vi "ref Begin.vi"(8 "error in":errorcluster) -> (0 "error out":errorcluster)   [LabVIEW 2020]
doc: "Called before other user functions, this VI is expected to open initial I/O refnums, load in file data, and do all program initialization. Notice that the <B>error out</B> terminal is simply used for data flow. Wiring it to other structures or subVIs ensures that this VI runs first."
uses:
  <vilib>/Rock Robotics/WPI/ThirdParty/Phoenix-LabVIEW/Motor Controller/Controls/CTRE_Phoenix_MotorControl_TalonFXMotorControllerConfigurables.ctl
  <vilib>/Rock Robotics/WPI/ThirdParty/Phoenix-LabVIEW/Motor Controller/Controls/CTRE_Phoenix_MotorControl_BaseConfigurables.ctl
  <vilib>/Rock Robotics/WPI/ThirdParty/Phoenix-LabVIEW/Motor Controller/Controls/CTRE_Phoenix_MotorControl_VelocityMeasurementPeriod.ctl
  <vilib>/Rock Robotics/WPI/ThirdParty/Phoenix-LabVIEW/Motor Controller/Controls/CTRE_Phoenix_MotorControl_SlotStructure.ctl
  <vilib>/Rock Robotics/WPI/ThirdParty/Phoenix-LabVIEW/Motor Controller/Controls/CTRE_Phoenix_MotorControl_FilterStruct.ctl
  <vilib>/Rock Robotics/WPI/ThirdParty/Phoenix-LabVIEW/Motor Controller/Controls/CTRE_Phoenix_MotorControl_RemoteSourceType.ctl
  <vilib>/Rock Robotics/WPI/ThirdParty/Phoenix-LabVIEW/Controls/CTRE_Phoenix_CustomParamConfiguration.ctl
  <vilib>/Rock Robotics/WPI/ThirdParty/Phoenix-LabVIEW/Motor Controller/Controls/CTRE_Phoenix_MotorControl_FeedbackDevice_TalonFX.ctl
  <vilib>/Rock Robotics/WPI/ThirdParty/Phoenix-LabVIEW/Motor Controller/Controls/CTRE_Phoenix_MotorControl_LimitSwitchNormal.ctl
  <vilib>/Rock Robotics/WPI/ThirdParty/Phoenix-LabVIEW/Motor Controller/Controls/CTRE_Phoenix_MotorControl_LimitSwitchSource_Local.ctl
  <vilib>/Rock Robotics/WPI/ThirdParty/Phoenix-LabVIEW/Motor Controller/Controls/CTRE_Phoenix_MotorControl_SupplyCurrentLimitConfiguration.ctl
  <vilib>/Rock Robotics/WPI/ThirdParty/Phoenix-LabVIEW/Motor Controller/Controls/CTRE_Phoenix_MotorControl_StatorCurrentLimitConfiguration.ctl
  <vilib>/Rock Robotics/WPI/ThirdParty/Phoenix-LabVIEW/Motor Controller/Controls/CTRE_Phoenix_MotorControl_MotorCommutation_TalonFX.ctl
  <vilib>/Rock Robotics/WPI/ThirdParty/Phoenix-LabVIEW/CANCoder/Controls/CTRE_Phoenix_CANcoder_AbsoluteSensorRange.ctl
  <vilib>/Rock Robotics/WPI/ThirdParty/Phoenix-LabVIEW/CANCoder/Controls/CTRE_Phoenix_CANcoder_SensorInitializationStrategy.ctl
  <vilib>/Rock Robotics/WPI/ThirdParty/Phoenix-LabVIEW/Motor Controller/Controls/CTRE_Phoenix_MotorControl_NeutralMode.ctl
  <vilib>/Rock Robotics/SystemInterfaces/DIO/FPGA_DIOChannel.ctl
  <vilib>/Rock Robotics/SystemInterfaces/DIO/FPGA_DIOPWMChannel.ctl
  <vilib>/Rock Robotics/WPI/Joystick/WPI_Joystick Info.ctl
  <vilib>/Rock Robotics/WPI/Joystick/WPI_JoystickHID Types.ctl
  <vilib>/Rock Robotics/WPI/Joystick/WPI_JoystickXBox Types.ctl
  <vilib>/Rock Robotics/WPI/Joystick/WPI_JoystickAxis Types.ctl
  <vilib>/Rock Robotics/WPI/Ultrasonic/WPI_UltrasonicRangeUnits.ctl
  <vilib>/Rock Robotics/WPI/Joystick/WPI_JoystickDeviceEnum.ctl
  <vilib>/Rock Robotics/WPI/DriverStation/WPI_DriverStationRobotMode2.ctl
  <vilib>/Rock Robotics/WPI/SafetyOutput/WPI_SafetyOutputConfigMenu.ctl
  <vilib>/Rock Robotics/SystemInterfaces/AI/FPGA_AIChannel.ctl
  <vilib>/Rock Robotics/SystemInterfaces/i2clib/i2c_bus.ctl
  <vilib>/Rock Robotics/Network Tables/NT Write String Array.vi
  Robot Global Data.vi
  <vilib>/Rock Robotics/WPI/RobotDrive/WPI_RobotDriveOpen2MotorWithExistingMotors.vi
  <vilib>/Rock Robotics/WPI/ThirdParty/REV Robotics/REVLib/Typedef/Spark MAX Motor Type.ctl
  <vilib>/Rock Robotics/WPI/ThirdParty/REV Robotics/REVLib/Typedef/Spark MAX Idle Mode.ctl
  <vilib>/Rock Robotics/Network Tables/NT Write Number.vi
  <vilib>/Rock Robotics/WPI/Ultrasonic/WPI_SonarSRF04DigitalOpen.vi
  <vilib>/Rock Robotics/WPI/Ultrasonic/WPI_SonarSRF04DigitalRefNum Registry Set.vi
  <vilib>/Rock Robotics/WPI/Ultrasonic/WPI_SonarSRF04DigitalGetRange.vi
  <vilib>/Rock Robotics/WPI/Counter/WPI_CounterDigitalInputToDigitalSource.vi
  <vilib>/Rock Robotics/Network Tables/NT Write Boolean.vi
  <vilib>/Rock Robotics/WPI/Counter/WPI_CounterOpen Gear Tooth Sensor Mode.vi
panel:
  in  "KICKER CAN ID 2":u8=10
  in  "Tab Control":T1(tab)=enum."SHOOTER"
  in  "drive wheel diameter (in)":dbl=6.0 format="%.3g"
  in  "drive gearbox ratio":dbl=10.71
  out "wheel circumference":dbl=18.84955592153876
  in  "MASTER LEFT DRIVE CAN ID":u8=2
  in  "LEFT MotorInverted":bool=TRUE
  in  "Motor Control Neutral Mode 3":T2=enum."Override to Coast"
  in  "CLIMBER COAST":T2=enum."Override to Brake"
  in  "CLIMBER LEFT CAN ID":u8=9
  in  "ARM LEFT CAN ID":u8=11
  in  "CLIMBER RIGHT CAN ID":u8=7
  in  "ARM RIGHT CAN ID":u8=15
  in  "Invert LEFT climber":bool
  in  "Invert arm actuators":bool
  in  "FALCON shooter config":T3={"Base Configurables"={"openLoopRamp"=0.0, "closedLoopRamp"=0.0, "peakOutputForward"=1.0, "peakOutputReverse"=-1.0, "nominalOutputForward"=0.0, "nominalOutputReverse"=0.0, "neutralDeadband"=0.04, "voltageCompSaturation"=0.0, "voltageMeasurementFilter"=32, "velocityMeasurementPeriod"=100, "velocityMeasurementWindow"=64, "forwardSoftLimitThreshold"=0, "reverseSoftLimitThreshold"=0, "forwardSoftLimitEnable"=FALSE, "reverseSoftLimitEnable"=FALSE, "slot0"={"P"=0.0, "I"=0.0, "D"=0.0, "F"=0.0, "integralZone"=0.0, "allowableClosedLoopError"=0, "maxIntegralAccumulator"=0.0, "closedLoopPeakOutput"=1.0, "closedLoopPeriod"=1}, "slot1"={"P"=0.0, "I"=0.0, "D"=0.0, "F"=0.0, "integralZone"=0.0, "allowableClosedLoopError"=0, "maxIntegralAccumulator"=0.0, "closedLoopPeakOutput"=1.0, "closedLoopPeriod"=1}, "slot2"={"P"=0.0, "I"=0.0, "D"=0.0, "F"=0.0, "integralZone"=0.0, "allowableClosedLoopError"=0, "maxIntegralAccumulator"=0.0, "closedLoopPeakOutput"=1.0, "closedLoopPeriod"=1}, "slot3"={"P"=0.0, "I"=0.0, "D"=0.0, "F"=0.0, "integralZone"=0.0, "allowableClosedLoopError"=0, "maxIntegralAccumulator"=0.0, "closedLoopPeakOutput"=1.0, "closedLoopPeriod"=1}, "auxPIDPolarity"=FALSE, "remoteFilter0"={"remoteSensorDeviceID"=0, "remoteSensorSource"=enum."Off"}, "remoteFilter1"={"remoteSensorDeviceID"=0, "remoteSensorSource"=enum."Off"}, "motionCruiseVelocity"=0, "motionAcceleration"=0, "motionProfileTrajectoryPeriod"=0, "feedbackNotContinuous"=FALSE, "remoteSensorClosedLoopDisableNeutralOnLOS"=FALSE, "clearPositionOnLimitF"=FALSE, "clearPositionOnLimitR"=FALSE, "clearPositionOnQuadIdx"=FALSE, "limitSwitchDisableNeutralOnLOS"=FALSE, "softLimitDisableNeutralOnLOS"=FALSE, "pulseWidthPeriod_EdgesPerRot"=1, "pulseWidthPeriod_FilterWindowSz"=1, "customParam"={"customParam0"=0, "customParam1"=0}, "trajectoryInterpolationEnable"=TRUE}, "primaryPID"={"selectedFeedbackCoefficient"=1.0, "selectedFeedbackSensor"=1}, "auxiliaryPID"={"selectedFeedbackCoefficient"=1.0, "selectedFeedbackSensor"=1}, "forwardLimitSwitchNormal"=enum."Normally Open", "reverseLimitSwitchNormal"=enum."Normally Open", "forwardLimitSwitchDeviceID"=0, "reverseLimitSwitchDeviceID"=0, "forwardLimitSwitchSource"=enum."Feedback Connector", "reverseLimitSwitchSource"=enum."Feedback Connector", "sum0Term"=1, "sum1Term"=1, "diff0Term"=1, "diff1Term"=1, "Supply Current Limit Configuration"={"Enable?"=FALSE, "Current Limit"=0.0, "Threshold Current"=0.0, "Threshold Time"=0.0}, "Stator Current Limit Configuration"={"Enable?"=FALSE, "Current Limit"=0.0, "Threshold Current"=0.0, "Threshold Time"=0.0}, "Motor Commutation"=enum."Trapezoidal", "Absolute Sensor Range"=enum."Unsigned [0 to 360)", "Integrated Sensor Offset (Degrees)"=0.0, "Sensor Initialization Strategy"=enum."Boot To Zero"} {"diff1Term" items=["Integrated Sensor"=1, "Sensor Sum (S0 + S1)"=9, "Sensor Difference (D0 - D1)"=10, "Remote Source 0"=11, "Remote Source 1"=12, "None"=14, "Software Emulated"=15]; "diff0Term" items=["Integrated Sensor"=1, "Sensor Sum (S0 + S1)"=9, "Sensor Difference (D0 - D1)"=10, "Remote Source 0"=11, "Remote Source 1"=12, "None"=14, "Software Emulated"=15]; "sum1Term" items=["Integrated Sensor"=1, "Sensor Sum (S0 + S1)"=9, "Sensor Difference (D0 - D1)"=10, "Remote Source 0"=11, "Remote Source 1"=12, "None"=14, "Software Emulated"=15]; "sum0Term" items=["Integrated Sensor"=1, "Sensor Sum (S0 + S1)"=9, "Sensor Difference (D0 - D1)"=10, "Remote Source 0"=11, "Remote Source 1"=12, "None"=14, "Software Emulated"=15]; "auxiliaryPID"."selectedFeedbackSensor" items=["Integrated Sensor"=1, "Sensor Sum (S0 + S1)"=9, "Sensor Difference (D0 - D1)"=10, "Remote Source 0"=11, "Remote Source 1"=12, "None"=14, "Software Emulated"=15]; "primaryPID"."selectedFeedbackSensor" items=["Integrated Sensor"=1, "Sensor Sum (S0 + S1)"=9, "Sensor Difference (D0 - D1)"=10, "Remote Source 0"=11, "Remote Source 1"=12, "None"=14, "Software Emulated"=15]; "Base Configurables"."velocityMeasurementPeriod" items=["Period_1ms"=1, "Period_2ms"=2, "Period_5ms"=5, "Period_10ms"=10, "Period_20ms"=20, "Period_25ms"=25, "Period_50ms"=50, "Period_100ms"=100]}
  in  "Motor Control Neutral Mode 2":T2=enum."Override to Brake"
  in  "SHOOTER CAN ID":u8=8
  in  "KICKER CAN ID":u8=21
  in  "KICKER COUNT DIO":T18
  in  "Sonars":T20(array[cluster])=[{"Sonar refnum name"="BALL1", "Ping DIO Channel"=enum."DIO 2", "Echo DIO Channel"=enum."DIO 3", "Range Units"=enum."inches"}, {"Sonar refnum name"="BALL2", "Ping DIO Channel"=enum."DIO 4", "Echo DIO Channel"=enum."DIO 5", "Range Units"=enum."inches"}]
  in  "Color Define":T21(array[cluster])
  out "Joystick INFO":T22[](array[typedef])
  in  "Joysticks":T27(array[cluster])=[{"JoystickDevice"=enum."USB 0", "refnum name"="Joystick 0"}, {"JoystickDevice"=enum."USB 1", "refnum name"="Joystick LEFT"}, {"JoystickDevice"=enum."USB 2", "refnum name"="Joystick RIGHT"}]
  in  "Power Distribution (def)":u8
  in  "Clear Sticky Faults":bool
  out "Channel Faults":bool[](array[boolean])
  out "Faults":T28
  out "Sticky Faults":T29
  out "error out 2":errorcluster={"status"=TRUE, "code"=-44087, "source"="NetComm_CAN_Receive.vi:5470010<APPEND>\n\n<b>Complete call chain:</b>\n     NetComm_CAN_Receive.vi:5470010\n     WPI_CAN_PDHReceive.vi\n     WPI_Power Get PD Faults.vi\n     Begin.vi\n     Robot Main.vi"}
  in  "TILT zero":u16=68
  in  "TILT Range":u16=170
  in  "PAN zero":u16=85
  in  "TILT  PWM Channel":T30=enum."PWM 1"
  in  "PAN Range":u16=170
  in  "PAN PWM Channel":T30
  # "Sum and Diff terms are ways to select more than one sensor as a feedback device. \n Sum 0 is the first feedback device to be used for the Sum term.\n Sum 1 is the feedback device to be added to Sum 0 for the Sum term.\n Diff 0 and Diff 1 work in a similar manner."
  # "These are only applicable\nif using a remote limit switch.\n\nLocal limit switches/no limit\nswitches do not use this."
  # "Current is below Current Limit AND\n\n(Requested output is weaker** than applied motor\noutput OR is in the opposite direction).\n/\nMotor output is set to requested output."
  # "Current is above Threshold Current for Threshold Time\n/\nReduce motor output (towards neutral)."
  # "Current is below Current Limit.\n/\nRamp motor output towards requested output."
  # "Current is above Current Limit.\n/\nReduce motor output (towards neutral)."
  # "*If the configured Peak Threshold is less than the Continuous Threshold, the applied Peak Threshold is set equal to the Configured Continuous Threshold in firmware.\n** Both requested output and applied motor output are in the same direction, and requested output is closer to neutral."
  # "False: Primary Output = PID[0] + PID[1]  ---  Auxiliary Output = PID[0] - PID[1]\nTrue:  Primary Output = PID[0] - PID[1] --- Auxiliary Output = PID[0] + PID[1]"
  # "Enable the motion profile executor to perform linear interpolation between profile points.  Defaults to True."
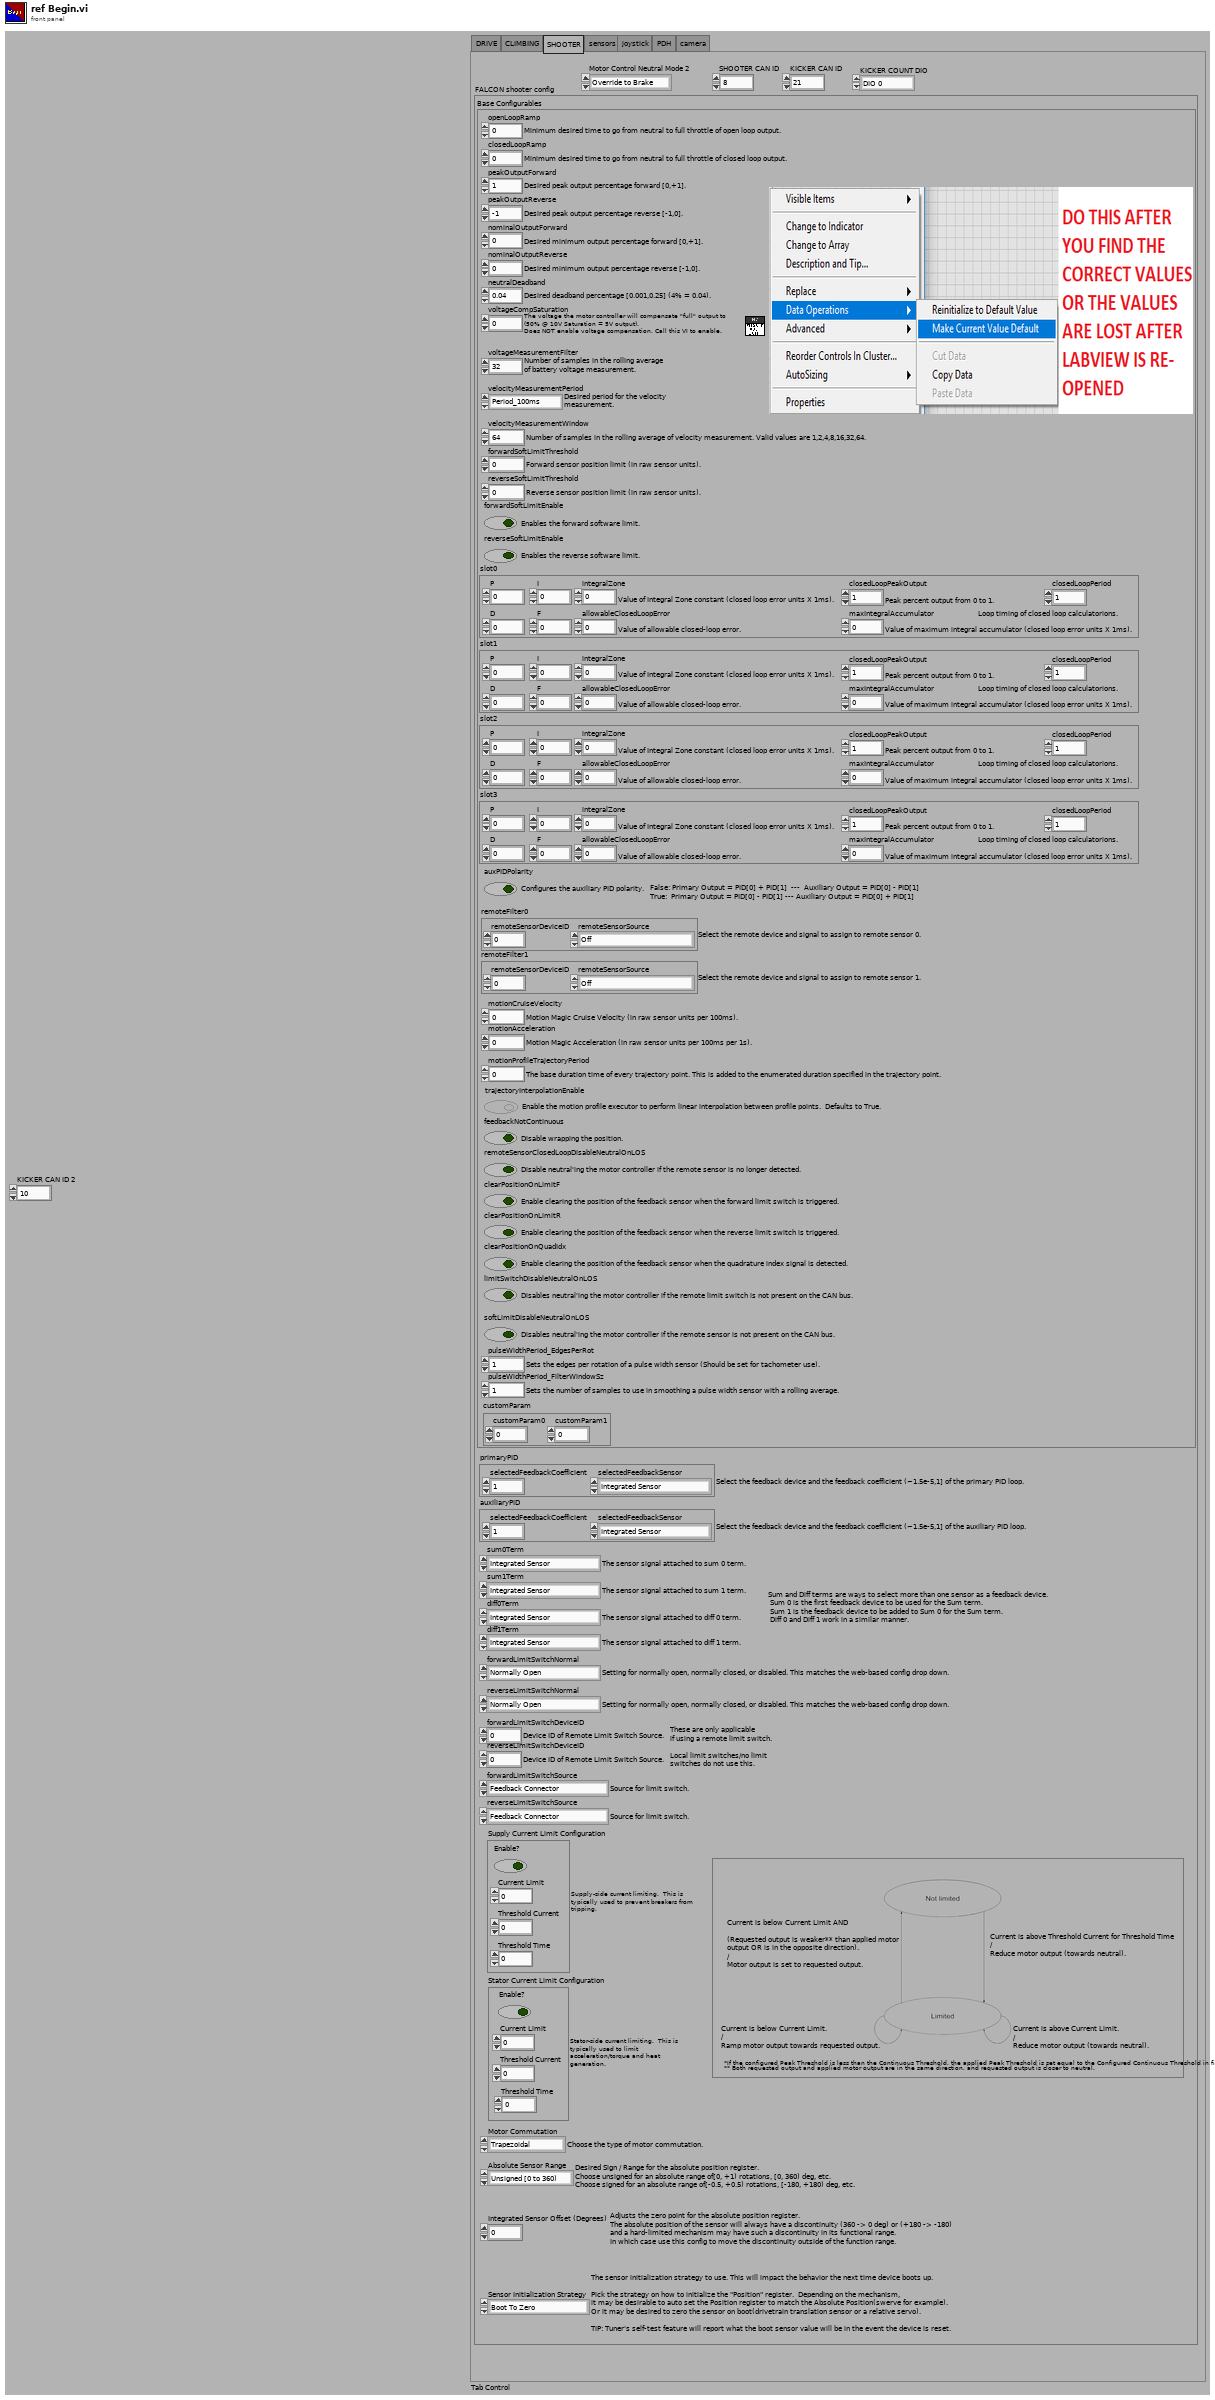
[diagram p1: front panel]
types:
  T1 = enum32{"DRIVE", "CLIMBING", "SHOOTER", "sensors", "joystick", "PDH", "camera"}
  T2 = typedef "CTRE_Phoenix_MotorControl_NeutralMode.ctl" = enum8{"EEPROMSetting", "Override to Coast", "Override to Brake"}
  T3 = typedef "CTRE_Phoenix_MotorControl_TalonFXMotorControllerConfigurables.ctl" = cluster{"Base Configurables":T4, "primaryPID":cluster{"selectedFeedbackCoefficient":dbl, "selectedFeedbackSensor":T10}, "auxiliaryPID":cluster{"selectedFeedbackCoefficient":dbl, "selectedFeedbackSensor":T10}, "forwardLimitSwitchNormal":T11, "reverseLimitSwitchNormal":T11, "forwardLimitSwitchDeviceID":i32, "reverseLimitSwitchDeviceID":i32, "forwardLimitSwitchSource":T12, "reverseLimitSwitchSource":T12, "sum0Term":T10, "sum1Term":T10, "diff0Term":T10, "diff1Term":T10, "Supply Current Limit Configuration":T13, "Stator Current Limit Configuration":T14, "Motor Commutation":T15, "Absolute Sensor Range":T16, "Integrated Sensor Offset (Degrees)":dbl, "Sensor Initialization Strategy":T17}
  T4 = typedef "CTRE_Phoenix_MotorControl_BaseConfigurables.ctl" = cluster{"openLoopRamp":dbl, "closedLoopRamp":dbl, "peakOutputForward":dbl, "peakOutputReverse":dbl, "nominalOutputForward":dbl, "nominalOutputReverse":dbl, "neutralDeadband":dbl, "voltageCompSaturation":dbl, "voltageMeasurementFilter":i32, "velocityMeasurementPeriod":T5, "velocityMeasurementWindow":i32, "forwardSoftLimitThreshold":i32, "reverseSoftLimitThreshold":i32, "forwardSoftLimitEnable":bool, "reverseSoftLimitEnable":bool, "slot0":T6, "slot1":T6, "slot2":T6, "slot3":T6, "auxPIDPolarity":bool, "remoteFilter0":T7, "remoteFilter1":T7, "motionCruiseVelocity":i32, "motionAcceleration":i32, "motionProfileTrajectoryPeriod":i32, "feedbackNotContinuous":bool, "remoteSensorClosedLoopDisableNeutralOnLOS":bool, "clearPositionOnLimitF":bool, "clearPositionOnLimitR":bool, "clearPositionOnQuadIdx":bool, "limitSwitchDisableNeutralOnLOS":bool, "softLimitDisableNeutralOnLOS":bool, "pulseWidthPeriod_EdgesPerRot":i32, "pulseWidthPeriod_FilterWindowSz":i32, "customParam":T9, "trajectoryInterpolationEnable":bool}
  T5 = typedef "CTRE_Phoenix_MotorControl_VelocityMeasurementPeriod.ctl" = u16
  T6 = typedef "CTRE_Phoenix_MotorControl_SlotStructure.ctl" = cluster{"P":dbl, "I":dbl, "D":dbl, "F":dbl, "integralZone":dbl, "allowableClosedLoopError":i32, "maxIntegralAccumulator":dbl, "closedLoopPeakOutput":dbl, "closedLoopPeriod":i32}
  T7 = typedef "CTRE_Phoenix_MotorControl_FilterStruct.ctl" = cluster{"remoteSensorDeviceID":u8, "remoteSensorSource":T8}
  T8 = typedef "CTRE_Phoenix_MotorControl_RemoteSourceType.ctl" = enum16{"Off", "Talon SRX Selected Sensor", "Pigeon IMU Yaw", "Pigeon IMU Pitch", "Pigeon IMU Roll", "CANifier Quadrature", "CANifier PWM Input 0", "CANifier PWM Input 1", "CANifier PWM Input 2", "CANifier PWM Input 3", "Gadgeteer Pigeon Yaw", "Gadgeteer Pigeon Pitch", "Gadgeteer Pigeon Roll", "CANCoder"}
  T9 = typedef "CTRE_Phoenix_CustomParamConfiguration.ctl" = cluster{"customParam0":i32, "customParam1":i32}
  T10 = typedef "CTRE_Phoenix_MotorControl_FeedbackDevice_TalonFX.ctl" = i8
  T11 = typedef "CTRE_Phoenix_MotorControl_LimitSwitchNormal.ctl" = enum16{"Normally Open", "Normally Closed", "Disabled"}
  T12 = typedef "CTRE_Phoenix_MotorControl_LimitSwitchSource_Local.ctl" = enum16{"Feedback Connector", "Remote Talon SRX", "Remote CANifier", "Deactivated"}
  T13 = typedef "CTRE_Phoenix_MotorControl_SupplyCurrentLimitConfiguration.ctl" = cluster{"Enable?":bool, "Current Limit":dbl, "Threshold Current":dbl, "Threshold Time":dbl}
  T14 = typedef "CTRE_Phoenix_MotorControl_StatorCurrentLimitConfiguration.ctl" = cluster{"Enable?":bool, "Current Limit":dbl, "Threshold Current":dbl, "Threshold Time":dbl}
  T15 = typedef "CTRE_Phoenix_MotorControl_MotorCommutation_TalonFX.ctl" = enum16{"Trapezoidal"}
  T16 = typedef "CTRE_Phoenix_CANcoder_AbsoluteSensorRange.ctl" = enum16{"Unsigned [0 to 360)", "Signed [-180 to +180)"}
  T17 = typedef "CTRE_Phoenix_CANcoder_SensorInitializationStrategy.ctl" = enum16{"Boot To Zero", "Boot To Absolute Position"}
  T18 = typedef "FPGA_DIOChannel.ctl" = enum8{"DIO 0", "DIO 1", "DIO 2", "DIO 3", "DIO 4", "DIO 5", "DIO 6", "DIO 7", "DIO 8", "DIO 9", "DIO MXP 0", "DIO MXP 1", "DIO MXP 2", "DIO MXP 3", "DIO MXP 4", "DIO MXP 5", "DIO MXP 6", "DIO MXP 7", "DIO MXP 8", "DIO MXP 9", "DIO MXP 10", "DIO MXP 11", "DIO MXP 12", "DIO MXP 13", "DIO MXP 14", "DIO MXP 15", "SPI Port CS1", "SPI Port CS2", "SPI Port CS3", "SPI Port MISO", "SPI Port MOSI", "Invalid"}
  T19 = typedef "WPI_UltrasonicRangeUnits.ctl" = enum16{"inches", "mm"}
  T20 = cluster{"Sonar refnum name":string, "Ping DIO Channel":T18, "Echo DIO Channel":T18, "Range Units":T19}[]
  T21 = cluster{"Name":string, "Color":cluster{"R":dbl, "G":dbl, "B":dbl}}[]
  T22 = typedef "WPI_Joystick Info.ctl" = cluster{"Device Name":string, "HID Type":T23, "XBox Type":T24, "Axes Count":i32, "Axes Types":T25[], "Button Count":i32, "POV Count":i32}
  T23 = typedef "WPI_JoystickHID Types.ctl" = enum16{"Not HID", "HID Joystick", "HID Gamepad", "HID Driving Wheel", "HID Flightstick", "HID First Person"}
  T24 = typedef "WPI_JoystickXBox Types.ctl" = enum16{"Not XBox", "XBox Unknown", "XBox Gamepad", "XBox Wheel", "XBox Arcade Stick", "XBox Flight Stick", "XBox Dance Pad", "XBox Guitar", "XBox Drum Kit", "XBox Arcade Pad"}
  T25 = typedef "WPI_JoystickAxis Types.ctl" = enum16{"X Axis", "Y Axis", "Z Axis", "RxAxis", "RyAxis", "RzAxis", "Slider", "POV", "None", "L X Axis", "L Y Axis", "L Trigger", "R Trigger", "R X Axis", "R Y Axis"}
  T26 = typedef "WPI_JoystickDeviceEnum.ctl" = enum16{"USB 0", "USB 1", "USB 2", "USB 3", "USB 4", "USB 5"}
  T27 = cluster{"JoystickDevice":T26, "refnum name":string}[]
  T28 = cluster{"Battery Voltage Fault":bool, "Hardware Fault":bool, "CAN Warning Fault":bool, "Temperature Fault":bool}
  T29 = cluster{"Brownout":bool, "CAN Warning":bool, "Can Bus Off":bool, "Hardware Fault":bool, "Firmware Fault":bool, "CH20 Brownout":bool, "CH21 Brownout":bool, "CH22 Brownout":bool, "CH23 Brownout":bool, "Has Reset":bool}
  T30 = typedef "FPGA_DIOPWMChannel.ctl" = enum8{"PWM 0", "PWM 1", "PWM 2", "PWM 3", "PWM 4", "PWM 5", "PWM 6", "PWM 7", "PWM 8", "PWM 9", "PWM MXP 0", "PWM MXP 1", "PWM MXP 2", "PWM MXP 3", "PWM MXP 4", "PWM MXP 5", "PWM MXP 6", "PWM MXP 7", "PWM MXP 8", "PWM MXP 9", "Invalid"}
  T31 = typedef "WPI_ServoDeviceRef.ctl" = cluster{"DeviceStatus":errorcluster, "PWM Channel":T30, "DeadBand":T32}
  T32 = typedef "WPI_PWMDeadband.ctl" = cluster{"Name":string, "maxPositivePwm":i32, "minPositivePwm":i32, "centerPwm":i32, "maxNegativePwm":i32, "minNegativePwm":i32, "angularRange":u16}
  T33 = typedef "WPI_MotorControlDeviceRef.ctl" = cluster{"DeviceStatus":errorcluster, "Type":T34, "PWM":cluster{"PWM Channel":T30, "DeadBand":T32}, "CAN":cluster{"Device Number":u8, "SetOutput VI Ref":variant, "GetOutput VI Ref":variant, "Enable VI Ref":variant, "Disable VI Ref":variant, "Data":variant}, "Invert":bool, "DIO PWM":cluster{"PWM \"Enable\" Channel":T30, "DIOChannel":T18, "PWM Rate":dbl}}
  T34 = typedef "WPI_MotorControlType.ctl" = enum16{"PWM", "CAN", "DIO PWM"}
  T35 = typedef "WPI_DriverStationRobotMode2.ctl" = enum16{"Autonomous Disabled", "Autonomous Enabled", "Teleop Disabled", "Teleop Enabled", "Disconnected", "Finish", "Test Disabled", "Test Enabled", "Emergency Stopped"}
  T36 = typedef "WPI_SafetyOutputConfigMenu.ctl" = enum16{"Enable", "Disable"}
  T37 = typedef "WPI_RobotDriveDevRef.ctl" = cluster{"DevStatus":errorcluster, "Motors[]":T33[], "Square Inputs":bool, "Max Output":dbl}
  T38 = typedef "Spark MAX Idle Mode.ctl" = enum16{"Coast", "Brake"}
  T39 = typedef "Spark MAX Motor Type.ctl" = enum16{"Brushed", "Brushless"}
  T40 = typedef "WPI_DigitalInputDevRef.ctl" = cluster{"DevStatus":errorcluster, "DIO Channel":T18}
  T41 = typedef "FPGA_CounterEncoderSourceConvertionLVSourceType.ctl" = cluster{"DevStatus":errorcluster, "AnalogTriggerMode?":bool, "DigitalMode":cluster{"DIO Channel":T42}, "AnalogTriggerMode":cluster{"AnalogTriggerIndex":T43, "OutputType":T44}}
  T42 = typedef "FPGA_DIODigitalSourceChannel.ctl" = enum8{"DIO 0", "DIO 1", "DIO 2", "DIO 3", "DIO 4", "DIO 5", "DIO 6", "DIO 7", "DIO 8", "DIO 9", "DIO MXP 0", "DIO MXP 1", "DIO MXP 2", "DIO MXP 3", "DIO MXP 4", "DIO MXP 5", "DIO MXP 6", "DIO MXP 7", "DIO MXP 8", "DIO MXP 9", "DIO MXP 10", "DIO MXP 11", "DIO MXP 12", "DIO MXP 13", "DIO MXP 14", "DIO MXP 15", "SPI Port CS1", "SPI Port CS2", "SPI Port CS3", "SPI Port MISO", "SPI Port MOSI", "Disabled"}
  T43 = typedef "FPGA_AnalogTriggerIndex.ctl" = enum8{"Trig 0", "Trig 1", "Trig 2", "Trig 3", "Trig 4", "Trig 5", "Trig 6", "Trig 7", "Invalid"}
  T44 = typedef "FPGA_AnalogTriggerOutType.ctl" = enum16{"InWindow", "TriggerState", "Rising", "Falling"}
  T45 = typedef "WPI_CounterDevRef.ctl" = cluster{"DevStatus":errorcluster, "CntIndex":T46}
  T46 = typedef "FPGA_CounterCtrSystemIndex.ctl" = enum8{"Ctr 0", "Ctr 1", "Ctr 2", "Ctr 3", "Ctr 4", "Ctr 5", "Ctr 6", "Ctr 7", "Invalid"}
  T47 = typedef "i2c_bus.ctl" = enum16{"I2C On-Board", "I2C MXP", "Invalid"}
  T48 = typedef "WPI_UltrasonicDeviceRef.ctl" = cluster{"DevStatus":errorcluster, "Ping Channel":T18, "Echo Channel":T18, "CntIndex":T46}
  T49 = typedef "Color Sensor V3 DevRef.ctl" = cluster{"I2CDevRef":T50}
  T50 = typedef "WPI_I2CDevRef.ctl" = cluster{"DevStatus":errorcluster, "Device Address":u8, "Handle":i32, "I2C Bus":T47}
  T51 = typedef "WPI_JoystickDevRef.ctl" = cluster{"Device":T26}
  T52 = typedef "FPGA_AIChannel.ctl" = enum8{"AI 0", "AI 1", "AI 2", "AI 3", "AI MXP 0", "AI MXP 1", "AI MXP 2", "AI MXP 3", "Invalid"}
  T53 = typedef "WPI_AnalogChannelDevRef.ctl" = cluster{"DevStatus":errorcluster, "Analog Channel":T52}
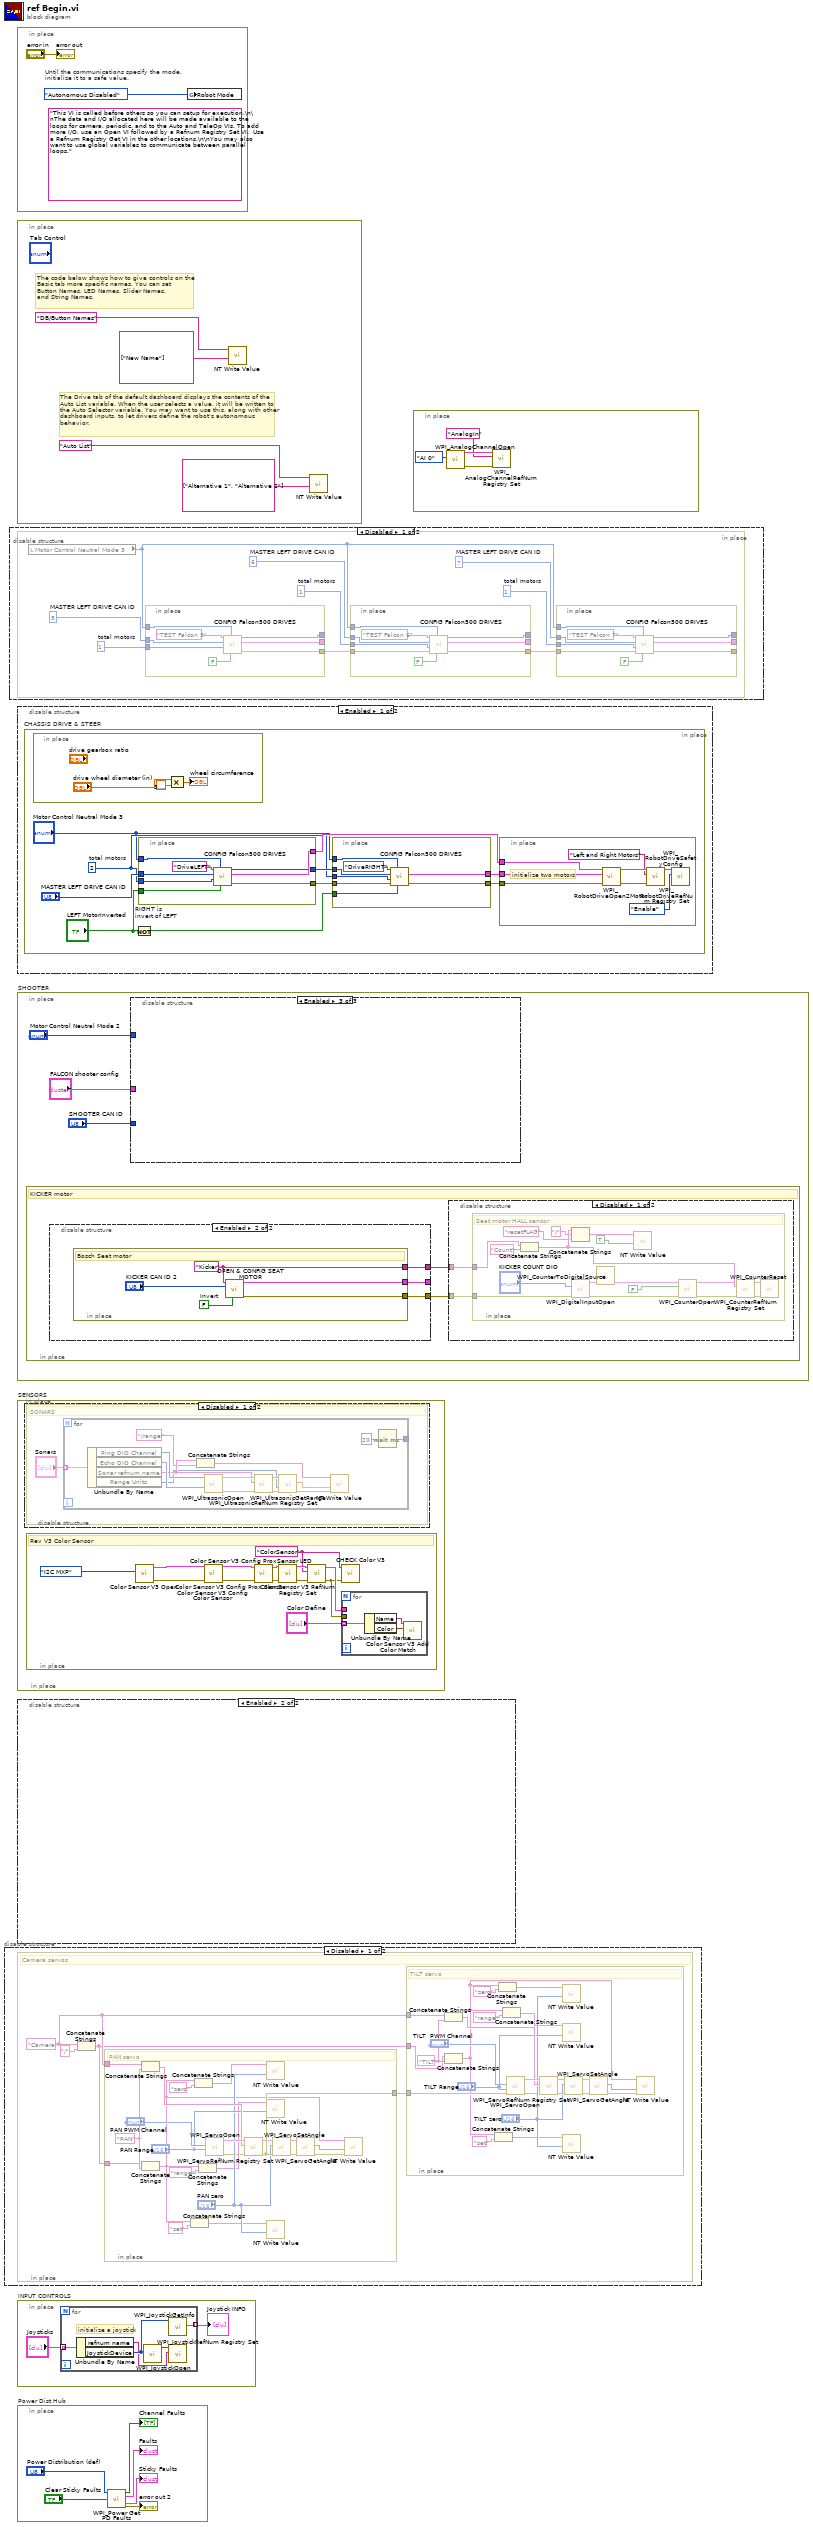
[diagram p0: block diagram]
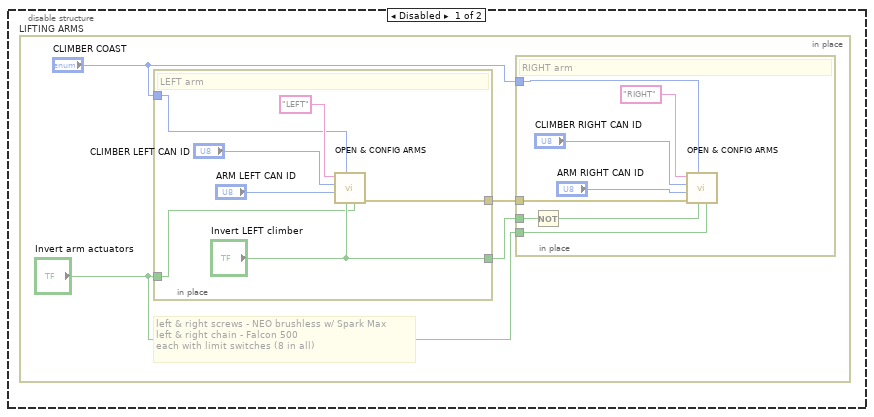
[diagram p5: hidden frame]
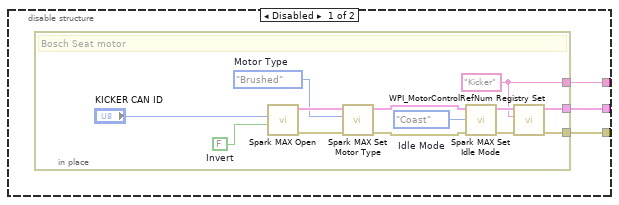
[diagram p7: hidden frame]
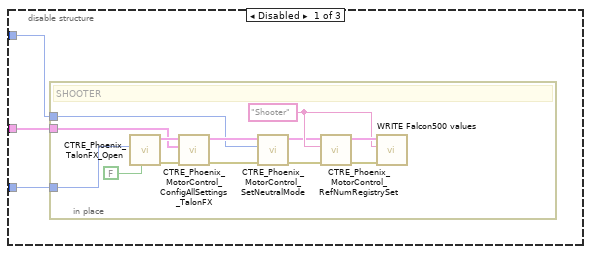
[diagram p8: hidden frame]
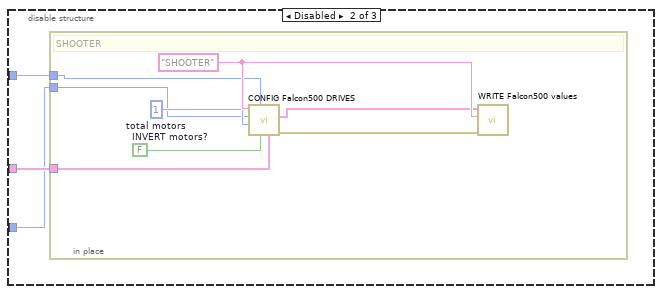
[diagram p9: hidden frame]
diagram:
  n1 = disable-structure shown="Disabled" {
    frame Disabled {
      n2 = in-place {
        w3 = "Camera" ("refnum name")
        # "Camera servos"
        n3 = Concatenate Strings(w3, "/" ("string")) -> (w1:string)
        n4 = in-place {
          in-place-border: [w23] -> w4
          in-place-border: w3 -> [w17]
          in-place-border: w1 -> [w16]
          w21 = "PAN" ("string")
          # "PAN servo"
          n5 = Concatenate Strings(w17, w21) -> (w24:string)
          n6 = Concatenate Strings(w16, w21) -> (w6:string)
          n7 = Concatenate Strings(w6, "set" ("Name")) -> (w7:string)
          n8 = Concatenate Strings(w6, "zero" ("string")) -> (w9:string)
          n9 = Concatenate Strings(w6, "range" ("string")) -> (w10:string)
          n10 = call <vilib>:"WPI_ServoOpen.vi"("Angular Range"="PAN Range", "PWM Channel"="PAN PWM Channel") -> ("error out"=w5:errorcluster, "ServoDeviceRef"=w26:T31)  [unwired: 8 in]
          n11 = call <vilib>:"WPI_ServoRefNum Registry Set.vi"("error in (no error)"=w5, "refnum name"=w24, "ServoDeviceRef"=w26) -> ("error out"=w23:errorcluster, "ServoDeviceRef"=w22:T31)  [unwired: 7 in]
          n12 = call-poly <vilib>:"NT Write Value.vi"("Numeric"="PAN zero", "Name"=w9) -> ()  [unwired: 9 in, 1 out]
          n13 = call-poly <vilib>:"NT Write Value.vi"("Numeric"="PAN Range", "Name"=w10) -> ()  [unwired: 9 in, 1 out]
          n14 = call-poly <vilib>:"NT Write Value.vi"("Numeric"="PAN zero", "Name"=w7) -> ()  [unwired: 9 in, 1 out]
          n15 = call <vilib>:"WPI_ServoSetAngle.vi"("error in (no error)"=w23, "Angle"="PAN zero", "ServoDeviceRef"=w22) -> ("error out"=w19:errorcluster, "ServoDeviceRef"=w20:T31)  [unwired: 7 in]
          n16 = call <vilib>:"WPI_ServoGetAngle.vi"("ServoDeviceRef"=w20, "error in (no error)"=w19) -> ("Angle"=w14:u16, "error out"=w15:errorcluster)  [unwired: 6 in, 1 out]
          n17 = call-poly <vilib>:"NT Write Value.vi"("error in"=w15, "Numeric"=w14, "Name"=w6) -> ()  [unwired: 8 in, 1 out]
        }
        n18 = in-place {
          in-place-border: w4 -> [w45]
          in-place-border: w3 -> [w43]
          in-place-border: w1 -> [w41]
          w42 = "TILT" ("string")
          # "TILT servo"
          n19 = Concatenate Strings(w43, w42) -> (w47:string)
          n20 = Concatenate Strings(w41, w42) -> (w28:string)
          n21 = Concatenate Strings(w28, "set" ("Name")) -> (w29:string)
          n22 = Concatenate Strings(w28, "zero" ("string")) -> (w31:string)
          n23 = Concatenate Strings(w28, "range" ("string")) -> (w32:string)
          n24 = call <vilib>:"WPI_ServoOpen.vi"("error in (no error)"=w45, "Angular Range"="TILT Range", "PWM Channel"="TILT  PWM Channel") -> ("error out"=w27:errorcluster, "ServoDeviceRef"=w49:T31)  [unwired: 7 in]
          n25 = call <vilib>:"WPI_ServoRefNum Registry Set.vi"("error in (no error)"=w27, "refnum name"=w47, "ServoDeviceRef"=w49) -> ("error out"=w46:errorcluster, "ServoDeviceRef"=w44:T31)  [unwired: 7 in]
          n26 = call-poly <vilib>:"NT Write Value.vi"("Numeric"="TILT zero", "Name"=w31) -> ()  [unwired: 9 in, 1 out]
          n27 = call-poly <vilib>:"NT Write Value.vi"("Numeric"="TILT Range", "Name"=w32) -> ()  [unwired: 9 in, 1 out]
          n28 = call-poly <vilib>:"NT Write Value.vi"("Numeric"="TILT zero", "Name"=w29) -> ()  [unwired: 9 in, 1 out]
          n29 = call <vilib>:"WPI_ServoSetAngle.vi"("error in (no error)"=w46, "Angle"="TILT zero", "ServoDeviceRef"=w44) -> ("error out"=w39:errorcluster, "ServoDeviceRef"=w40:T31)  [unwired: 7 in]
          n30 = call <vilib>:"WPI_ServoGetAngle.vi"("ServoDeviceRef"=w40, "error in (no error)"=w39) -> ("Angle"=w35:u16, "error out"=w36:errorcluster)  [unwired: 6 in, 1 out]
          n31 = call-poly <vilib>:"NT Write Value.vi"("error in"=w36, "Numeric"=w35, "Name"=w28) -> ()  [unwired: 8 in, 1 out]
        }
      }
    }
    frame Enabled {
    }
  }
  n32 = disable-structure shown="Disabled" {
    frame Disabled {
      n33 = in-place "In Place Element Structure" {
        w53 = u8 7  # MASTER LEFT DRIVE CAN ID
        w54 = 1  # total motors
        w55 = u8 6  # MASTER LEFT DRIVE CAN ID
        w56 = 1  # total motors
        w57 = 1  # total motors
        w58 = u8 5  # MASTER LEFT DRIVE CAN ID
        n34 = local read "Motor Control Neutral Mode 3"() -> (w50:T2)
        n35 = in-place {
          in-place-border: [w75] -> _
          in-place-border: w58 -> [w74]
          in-place-border: [w72] -> w52
          in-place-border: [w71] -> _
          in-place-border: w57 -> [w70]
          in-place-border: w50 -> [w69]
          n36 = call "CONFIG Falcon500 DRIVES.vi"("INVERT motors?"=FALSE, "Motor Control Neutral Mode"=w69, "total motors"=w70, "CAN ID for MASTER DRIVE"=w74, "MASTER DRIVE REF name"="TEST Falcon 5" ("refnum name")) -> ("error out"=w72:errorcluster, "PhoenixMotorControlDevRef"=w75:T33, "next CAN ID"=w71:u8)  [unwired: 4 in]
        }
        n37 = in-place {
          in-place-border: [w84] -> _
          in-place-border: w55 -> [w83]
          in-place-border: [w81] -> w51
          in-place-border: [w80] -> _
          in-place-border: w56 -> [w79]
          in-place-border: w50 -> [w78]
          in-place-border: w52 -> [w76]
          n38 = call "CONFIG Falcon500 DRIVES.vi"("INVERT motors?"=FALSE, "Motor Control Neutral Mode"=w78, "error in"=w76, "total motors"=w79, "CAN ID for MASTER DRIVE"=w83, "MASTER DRIVE REF name"="TEST Falcon 6" ("refnum name")) -> ("error out"=w81:errorcluster, "PhoenixMotorControlDevRef"=w84:T33, "next CAN ID"=w80:u8)  [unwired: 3 in]
        }
        n39 = in-place {
          in-place-border: [w67] -> _
          in-place-border: w53 -> [w66]
          in-place-border: [w64] -> _
          in-place-border: [w63] -> _
          in-place-border: w54 -> [w62]
          in-place-border: w50 -> [w61]
          in-place-border: w51 -> [w59]
          n40 = call "CONFIG Falcon500 DRIVES.vi"("INVERT motors?"=FALSE, "Motor Control Neutral Mode"=w61, "error in"=w59, "total motors"=w62, "CAN ID for MASTER DRIVE"=w66, "MASTER DRIVE REF name"="TEST Falcon 7" ("refnum name")) -> ("error out"=w64:errorcluster, "PhoenixMotorControlDevRef"=w67:T33, "next CAN ID"=w63:u8)  [unwired: 3 in]
        }
      }
    }
    frame Enabled {
    }
  }
  n41 = in-place {
    (unwired) "This VI is called before others so you can setup for execution.\n\nThe data and I/O allocated here will be made available to the loops for camera, periodic, and to the Auto and TeleOp VIs. To add more I/O, use an Open VI followed by a Refnum Registry Set VI.  Use a Refnum Registry Get VI in the other locations.\n\nYou may also want to use global variables to communicate between parallel loops."
    # "Until the communications specify the mode,\ninitialize it to a safe value."
    n42 = global write "Robot Global Data.vi" "Robot Mode"(WPI_DriverStationRobotMode2."Autonomous Disabled" ("Robot Mode")) -> ()
    "error out" <- "error in"
  }
  n43 = in-place {
    # "The Drive tab of the default dashboard displays the contents of the\nAuto List variable. When the user selects a value, it will be written to\nthe Auto Selector variable. You may want to use this, along with other\ndashboard inputs, to let drivers define the robot's autonomous\nbehavior."
    # "The code below shows how to give controls on the\nBasic tab more specific names. You can set\nButton Names, LED Names, Slider Names,\nand String Names."
    n44 = call-poly <vilib>:"NT Write Value.vi"("String Array"=string[] ["New Name"], "Name"="DB/Button Names") -> ()  [unwired: 9 in, 1 out]
    n45 = call-poly <vilib>:"NT Write Value.vi"("String Array"=string[] ["Alternative 1", "Alternative 2"], "Name"="Auto List") -> ()  [unwired: 9 in, 1 out]
  }
  n46 = disable-structure shown="Enabled" {
    frame Enabled {
      n47 = in-place "CHASSIS DRIVE & STEER" {
        w92 = 2  # total motors
        n48 = in-place {
          n49 = Multiply(x="drive wheel diameter (in)", y=3.141592653589793) -> (x*y=→"wheel circumference":dbl)
        }
        n50 = Not "RIGHT is\ninvert of LEFT"(x="LEFT MotorInverted") -> (.not. x?=w94:bool)
        n51 = in-place {
          in-place-border: [w108] -> w100
          in-place-border: "MASTER LEFT DRIVE CAN ID" -> [w107]
          in-place-border: "LEFT MotorInverted" -> [w106]
          in-place-border: [w104] -> w95
          in-place-border: [w103] -> w93
          in-place-border: w92 -> [w102]
          in-place-border: "Motor Control Neutral Mode 3" -> [w101]
          n52 = call "CONFIG Falcon500 DRIVES.vi"("INVERT motors?"=w106, "Motor Control Neutral Mode"=w101, "total motors"=w102, "CAN ID for MASTER DRIVE"=w107, "MASTER DRIVE REF name"="DriveLEFT" ("refnum name")) -> ("error out"=w104:errorcluster, "PhoenixMotorControlDevRef"=w108:T33, "next CAN ID"=w103:u8)  [unwired: 4 in]
        }
        n53 = in-place {
          in-place-border: [w116] -> w97
          in-place-border: [w115] -> w96
          in-place-border: w95 -> [w114]
          in-place-border: w94 -> [w113]
          in-place-border: w93 -> [w111]
          in-place-border: w92 -> [w110]
          in-place-border: "Motor Control Neutral Mode 3" -> [w109]
          n54 = call "CONFIG Falcon500 DRIVES.vi"("INVERT motors?"=w113, "Motor Control Neutral Mode"=w109, "error in"=w114, "total motors"=w110, "CAN ID for MASTER DRIVE"=w111, "MASTER DRIVE REF name"="DriveRIGHT" ("refnum name")) -> ("error out"=w115:errorcluster, "PhoenixMotorControlDevRef"=w116:T33)  [unwired: 3 in, 1 out]
        }
        n55 = in-place {
          in-place-border: w100 -> [w119]
          in-place-border: w97 -> [w118]
          in-place-border: w96 -> [w117]
          # "initialize two motors"
          n56 = call-poly <vilib>:"WPI_RobotDriveOpen2Motor.vi"("error in (no error)"=w117, "Right Motor Dev Ref"=w118, "Left Motor Dev Ref"=w119) -> ("error out"=w122:errorcluster, "RobotDriveDevRef"=w124:T37)  [unwired: 2 in, 5 out]
          n57 = call <vilib>:"WPI_RobotDriveRefNum Registry Set.vi"("error in (no error)"=w122, "refnum name"="Left and Right Motors", "RobotDriveDevRef"=w124) -> ("RobotDriveDevRef"=w121:T37)  [unwired: 1 in, 7 out]
          n58 = call <vilib>:"WPI_RobotDriveSafetyConfig.vi"("mode"=WPI_SafetyOutputConfigMenu."Enable", "RobotDriveDevRef"=w121) -> ()  [unwired: 8 in, 2 out]
        }
      }
    }
    frame Disabled {
    }
  }
  n59 = in-place "SHOOTER" {
    n60 = in-place {
      # "KICKER motor"
      n61 = disable-structure shown="Enabled" {
        disable-tunnel: [w154 w168] -> w132
        disable-tunnel: [w153 w169] -> w131
        disable-tunnel: [w152 w170] -> _
        frame Disabled {
          n62 = in-place {
            in-place-border: [w158] -> w154
            in-place-border: [w157] -> w153
            in-place-border: [w155] -> w152
            w156 = FALSE  # Invert
            w157 = "Kicker" ("refnum name")
            w161 = Spark_MAX_Idle_Mode."Coast"  # Idle Mode
            w164 = Spark_MAX_Motor_Type."Brushed"  # Motor Type
            # "Bosch Seat motor"
            n63 = call <vilib>:"Spark MAX Open.vi"("Invert"=w156, "Device Number"="KICKER CAN ID") -> ("error out"=w166:errorcluster, "MotorControlDeviceRef"=w165:T33)  [unwired: 8 in]
            n64 = call <vilib>:"Spark MAX Set Motor Type.vi"("error in (no error)"=w166, "Motor Type"=w164, "MotorControlDevRef"=w165) -> ("error out"=w163:errorcluster, "MotorControlDeviceRef"=w162:T33)  [unwired: 7 in]
            n65 = call <vilib>:"Spark MAX Set Idle Mode.vi"("error in (no error)"=w163, "Idle Mode"=w161, "MotorControlDeviceRef in"=w162) -> ("error out"=w160:errorcluster, "MotorControlDeviceRef out"=w159:T33)  [unwired: 7 in]
            n66 = call <vilib>:"WPI_MotorControlRefNum Registry Set.vi"("error in (no error)"=w160, "refnum name"=w157, "MotorControlDevRef"=w159) -> ("error out"=w158:errorcluster, "MotorControlDevRef"=w155:T33)  [unwired: 7 in]
          }
        }
        frame Enabled {
          n67 = in-place {
            in-place-border: [w174] -> w168
            in-place-border: [w173] -> w169
            in-place-border: [w172] -> w170
            w171 = FALSE  # Invert
            w173 = "Kicker" ("refnum name")
            # "Bosch Seat motor"
            n68 = call "OPEN & CONFIG SEAT MOTOR.vi"("Invert"=w171, "KICKER CAN ID in"="KICKER CAN ID 2", "refnum name"=w173) -> ("error out"=w174:errorcluster, "PhoenixMotorControlDevRef"=w172:T33)  [unwired: 7 in]
          }
        }
      }
      n69 = disable-structure shown="Disabled" {
        disable-tunnel: w132 -> [w134 _]
        disable-tunnel: w131 -> [w133 _]
        frame Disabled {
          n70 = in-place {
            in-place-border: w134 -> [w150]
            in-place-border: w133 -> [w149]
            # "Seat motor HALL sensor"
            n71 = Concatenate Strings(w149, "Count" ("refnum name")) -> (w147:string)
            n72 = Concatenate Strings(w147, "/" ("string"), "resetFLAG" ("string")) -> (w146:string)
            n73 = call <vilib>:"WPI_DigitalInputOpen.vi"("error in (no error)"=w150, "DIO Channel"="KICKER COUNT DIO") -> ("error out"=w140:errorcluster, "DigitalInputDevRef"=w141:T40)  [unwired: 8 in]
            n74 = call-poly <vilib>:"WPI_CounterToDigitalSource.vi"("DigitalInputDevRef"=w141) -> ("Digital Source"=w142:T41)  [unwired: 6 in]
            n75 = call-poly <vilib>:"NT Write Value.vi"("Boolean"=TRUE, "Name"=w146) -> ()  [unwired: 9 in, 1 out]
            n76 = call-poly <vilib>:"WPI_CounterOpen.vi"("error in (no error)"=w140, "Direction Sensitive"=FALSE, "Source"=w142) -> ("error out"=w138:errorcluster, "CounterDevRef"=w139:T45)  [unwired: 4 in, 3 out]
            n77 = call <vilib>:"WPI_CounterRefNum Registry Set.vi"("error in (no error)"=w138, "refnum name"=w147, "CounterDevRef"=w139) -> ("error out"=w137:errorcluster, "CounterDevRef"=w136:T45)  [unwired: 7 in]
            n78 = call <vilib>:"WPI_CounterReset.vi"("error in (no error)"=w137, "CounterDevRef in"=w136) -> ()  [unwired: 8 in, 2 out]
          }
        }
        frame Enabled {
        }
      }
    }
    n79 = disable-structure shown="Enabled" {
      disable-tunnel: "Motor Control Neutral Mode 2" -> [w178 w192 _]
      disable-tunnel: "FALCON shooter config" -> [w177 w194 _]
      disable-tunnel: "SHOOTER CAN ID" -> [w176 w193 _]
      frame Disabled {
        n80 = in-place {
          in-place-border: w178 -> [w181]
          in-place-border: w177 -> [w180]
          in-place-border: w176 -> [w179]
          w186 = "Shooter" ("refnum name")
          # "SHOOTER"
          n81 = call <vilib>:"CTRE_Phoenix_TalonFX_Open.vi"("Invert"=FALSE, "Device Number"=w179) -> ("error out"=w191:errorcluster, "PhoenixMotorControlDevRef"=w190:T33)  [unwired: 8 in]
          n82 = call <vilib>:"CTRE_Phoenix_MotorControl_ConfigAllSettings_TalonFX.vi"("error in (no error)"=w191, "Talon FX Configurables"=w180, "PhoenixMotorControlDevRef"=w190) -> ("error out"=w182:errorcluster, "PhoenixMotorControlDevRef"=w185:T33)  [unwired: 7 in]
          n83 = call <vilib>:"CTRE_Phoenix_MotorControl_SetNeutralMode.vi"("error in (no error)"=w182, "Motor Control Neutral Mode"=w181, "PhoenixMotorControlDevRef"=w185) -> ("error out"=w183:errorcluster, "PhoenixMotorControlDevRef"=w184:T33)  [unwired: 7 in]
          n84 = call <vilib>:"CTRE_Phoenix_MotorControl_RefNumRegistrySet.vi"("error in (no error)"=w183, "refnum name"=w186, "PhoenixMotorControlDevRef"=w184) -> ("error out"=w187:errorcluster, "PhoenixMotorControlDevRef"=w188:T33)  [unwired: 7 in]
          n85 = call "WRITE Falcon500 values.vi"("PhoenixMotorControlDevRef"=w188, "refnum name"=w186, "error in (no error)"=w187) -> ()  [unwired: 5 in, 2 out]
        }
      }
      frame Disabled {
        n86 = in-place {
          in-place-border: w194 -> [w202]
          in-place-border: w193 -> [w196]
          in-place-border: w192 -> [w195]
          w197 = 1  # total motors
          w201 = FALSE  # INVERT motors?
          w200 = "SHOOTER" ("refnum name")
          # "SHOOTER"
          n87 = call "CONFIG Falcon500 DRIVES.vi"("Talon FX Configurables"=w202, "INVERT motors?"=w201, "Motor Control Neutral Mode"=w195, "total motors"=w197, "CAN ID for MASTER DRIVE"=w196, "MASTER DRIVE REF name"=w200) -> ("error out"=w199:errorcluster, "PhoenixMotorControlDevRef"=w198:T33)  [unwired: 3 in, 1 out]
          n88 = call "WRITE Falcon500 values.vi"("PhoenixMotorControlDevRef"=w198, "refnum name"=w200, "error in (no error)"=w199) -> ()  [unwired: 5 in, 2 out]
        }
      }
      frame Enabled {
      }
    }
  }
  n89 = in-place "SENSORS" {
    n90 = disable-structure shown="Disabled" {
      frame Disabled {
        n91 = in-place {
          # "SONARS"
          n92 = for {
            tunnel: "Sonars" -> [w214] mode=indexing
            tunnel: [w204] -> _
            n93 = Unbundle By Name(w214) -> ("Ping DIO Channel"=w213:T18, "Echo DIO Channel"=w212:T18, "Sonar refnum name"=w211:string, "Range Units"=w208:T19)
            n94 = Concatenate Strings(w211, "/range" ("string")) -> (w210:string)
            n95 = call-poly <vilib>:"WPI_UltrasonicOpen.vi"("Echo DIO Channel"=w212, "Ping DIO Channel"=w213) -> ("error out"=w218:errorcluster, "UltrasonicDevRef"=w217:T48)  [unwired: 8 in]
            n96 = call-poly <vilib>:"WPI_UltrasonicRefNum Registry Set.vi"("error in (no error)"=w218, "refnum name"=w211, "SonarSRF04DevRef"=w217) -> ("error out"=w216:errorcluster, "SonarSRF04DevRef"=w215:T48)  [unwired: 7 in]
            n97 = call-poly <vilib>:"WPI_UltrasonicGetRange.vi"("error in (no error)"=w216, "Range Units"=w208, "UltrasonicDevRef"=w215) -> ("error out"=w207:errorcluster, "Distance"=w206:dbl)  [unwired: 6 in, 1 out]
            n98 = call-poly <vilib>:"NT Write Value.vi"("error in"=w207, "Numeric"=w206, "Name"=w210) -> ()  [unwired: 8 in, 1 out]
            n99 = Wait (ms)(milliseconds to wait=u32 20) -> (millisecond timer value=w204:u32)
          }
        }
      }
      frame Enabled {
      }
    }
    n100 = in-place "In Place Element Structure" {
      w220 = "ColorSensor" ("refnum name")
      # "Rev V3 Color Sensor"
      n101 = call <vilib>:"Color Sensor V3 Open.vi"("I2C Bus"=i2c_bus."I2C MXP") -> ("error out"=w230:errorcluster, "ColorSensorDevRef"=w231:T49)  [unwired: 9 in]
      n102 = call <vilib>:"Color Sensor V3 Config Color Sensor.vi"("ColorSensorDevRef"=w231, "error in (no error)"=w230) -> ("ColorSensorDevRef out"=w228:T49, "error out"=w229:errorcluster)  [unwired: 12 in]
      n103 = call <vilib>:"Color Sensor V3 Config Prox Sensor.vi"("error in (no error)"=w229, "ColorSensorDevRef"=w228) -> ("error out"=w226:errorcluster, "ColorSensorDevRef out"=w227:T49)  [unwired: 8 in]
      n104 = call <vilib>:"Color Sensor V3 Config ProxSensor LED.vi"("ColorSensorDevRef"=w227, "error in (no error)"=w226) -> ("ColorSensorDevRef out"=w224:T49, "error out"=w225:errorcluster)  [unwired: 12 in]
      n105 = call <vilib>:"Color Sensor V3 RefNum Registry Set.vi"("error in (no error)"=w225, "refnum name"=w220, "ColorSensorDevRef"=w224) -> ("error out"=w219:errorcluster, "ColorSensorDevRef out"=w221:T49)  [unwired: 7 in]
      n106 = call "CHECK Color V3.vi"("error in (no error)"=w219, "refnum name"=w220) -> ()  [unwired: 5 in, 5 out]
      n107 = for {
        tunnel: "Color Define" -> [w234] mode=indexing
        tunnel: w219 -> [_]
        tunnel: w221 -> [_]
        n108 = Unbundle By Name(w234) -> ("Name"=w233:string, "Color"=w232:cluster{"R":dbl, "G":dbl, "B":dbl})
        n109 = call <vilib>:"Color Sensor V3 Add Color Match.vi"("Color"=w232, "Name"=w233) -> ()  [unwired: 10 in]
      }
    }
  }
  n110 = disable-structure shown="Enabled" {
    frame Disabled {
      n111 = in-place "LIFTING ARMS" {
        # "left & right screws - NEO brushless w/ Spark Max\nleft & right chain - Falcon 500\neach with limit switches (8 in all)"
        n112 = in-place {
          in-place-border: "CLIMBER COAST" -> [w242]
          in-place-border: ["Invert LEFT climber"] -> w237
          in-place-border: "Invert arm actuators" -> [w240]
          in-place-border: [w239] -> w235
          # "LEFT arm"
          n113 = call "OPEN & CONFIG ARMS.vi"("Invert arm actuator?"=w240, "Invert climber?"="Invert LEFT climber", "CLIMBER COAST"=w242, "ARM CAN ID"="ARM LEFT CAN ID", "CLIMBER CAN ID"="CLIMBER LEFT CAN ID", "LEFT or RIGHT"="LEFT" ("refnum name")) -> ("error out"=w239:errorcluster)  [unwired: 5 in]
        }
        n114 = in-place {
          in-place-border: "CLIMBER COAST" -> [w250]
          in-place-border: w237 -> [w249]
          in-place-border: "Invert arm actuators" -> [w248]
          in-place-border: w235 -> [w247]
          # "RIGHT arm"
          n115 = Not(x=w249) -> (.not. x?=w246:bool)
          n116 = call "OPEN & CONFIG ARMS.vi"("Invert arm actuator?"=w248, "Invert climber?"=w246, "CLIMBER COAST"=w250, "error in (no error)"=w247, "ARM CAN ID"="ARM RIGHT CAN ID", "CLIMBER CAN ID"="CLIMBER RIGHT CAN ID", "LEFT or RIGHT"="RIGHT" ("refnum name")) -> ()  [unwired: 4 in, 1 out]
        }
      }
    }
    frame Enabled {
    }
  }
  n117 = in-place "INPUT CONTROLS" {
    n118 = for {
      tunnel: "Joysticks" -> [w259] mode=indexing
      tunnel: [w256] -> w254 mode=indexing
      # "initialize a joystick"
      n119 = Unbundle By Name(w259) -> ("refnum name"=w257:string, "JoystickDevice"=w258:T26)
      n120 = call <vilib>:"WPI_JoystickOpen.vi"("JoystickDevice"=w258) -> ("JoystickDevRef"=w260:T51)  [unwired: 10 in]
      n121 = call <vilib>:"WPI_JoystickGetInfo.vi"("JoystickDevice"=w258) -> ("Joystick Info"=w256:T22)  [unwired: 9 in, 1 out]
      n122 = call <vilib>:"WPI_JoystickRefNum Registry Set.vi"("refnum name"=w257, "JoystickDevRef"=w260) -> ()  [unwired: 8 in, 2 out]
    }
    "Joystick INFO" <- w254
  }
  n123 = in-place "Power Dist Hub" {
    n124 = call <vilib>:"WPI_Power Get PD Faults.vi"("Power Distribution (def)"="Power Distribution (def)", "Clear Sticky Faults"="Clear Sticky Faults") -> ("Channel Faults"=→"Channel Faults":bool[], "Faults"=→"Faults":T28, "Sticky Faults"=→"Sticky Faults":T29, "error out"=→"error out 2":errorcluster)  [unwired: 10 in]
  }
  n125 = in-place {
    n126 = call <vilib>:"WPI_AnalogChannelOpen.vi"("Analog Channel"=FPGA_AIChannel."AI 0") -> ("error out"=w270:errorcluster, "AIDeviceRef"=w269:T53)  [unwired: 9 in]
    n127 = call <vilib>:"WPI_AnalogChannelRefNum Registry Set.vi"("error in (no error)"=w270, "refnum name"="AnalogIn", "AIDeviceRef"=w269) -> ()  [unwired: 7 in, 2 out]
  }
